vi "ex_getDaqmxChannelPropertiesCore.vi"(6 "channel props":T1[](array[typedef]), 7 "String":string, 8 "error in (no error)":errorcluster, 9 "property names (manual)":string[](array[string]), 10 "property names (autofill)":string[](array[string]), 11 "DAQmx Task":refnum<k21>) -> (0 "error out":errorcluster, 1 "Array 2":string[][](array[string]), 3 "Array":T1[][](array[typedef]))   [LabVIEW 2017]
uses:
  <vilib>/express/express shared/ex_EditUserDefinedProperties/usiDataType.ctl
  <vilib>/express/express shared/ExFile.llb/ex_TdmProperty.ctl
  <resource>/objmgr/daqmx.rc
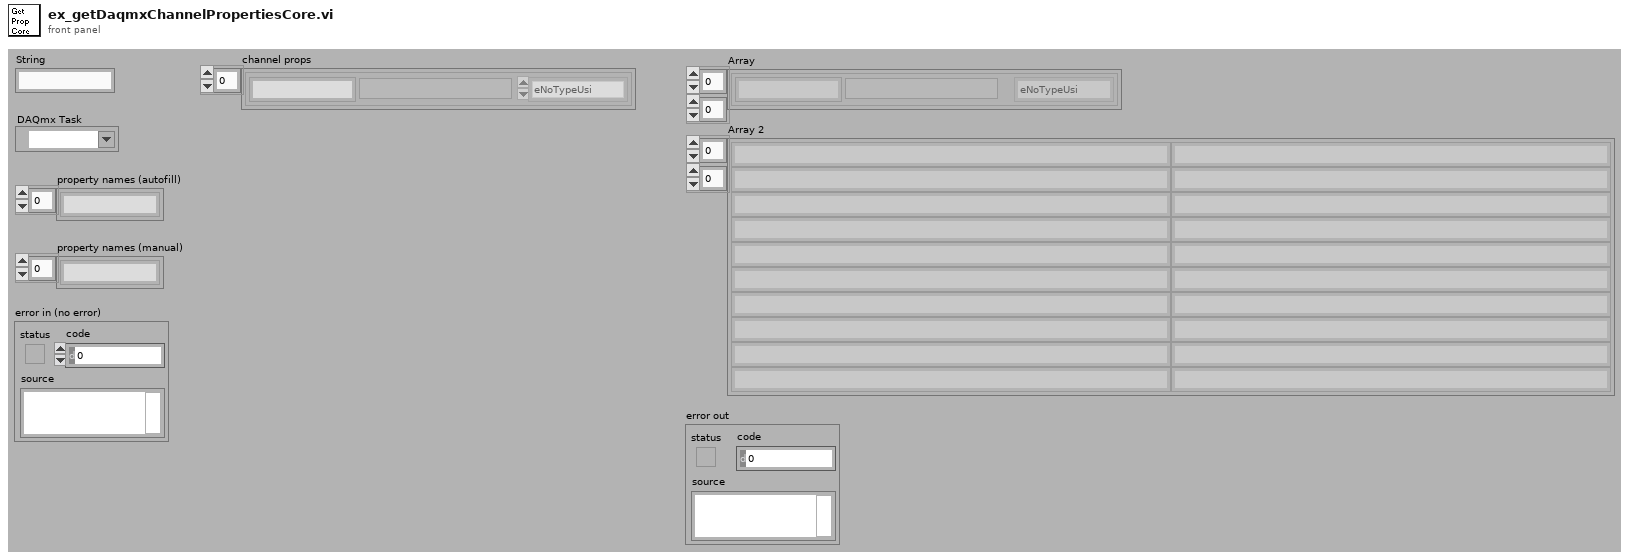
[diagram p1: front panel]
types:
  T1 = typedef "ex_TdmProperty.ctl" = cluster{"Name":string, "Type":T2, "Value":variant}
  T2 = typedef "usiDataType.ctl" = enum16{"eNoTypeUsi", "eInt8Usi", "eInt16Usi", "eInt32Usi", "eInt64Usi", "eUInt8Usi", "eUInt16Usi", "eUInt32Usi", "eUInt64Usi", "eFloat32Usi", "eFloat64Usi", "- 0", "- 1", "- 2", "- 3", "- 4", "- 5", "- 6", "- 7", "- 8", "- 9", "eString8Usi", "eString16Usi", "eStringUsi", "eEnumUsi", "- 10", "- 11", "- 12", "- 13", "- 14", "eTimeUsi", "- 15", "- 16", "- 17", "- 18", "- 19", "- 20", "- 21", "- 22", "- 23", "eInstanceUsi", "eStoreUsi"}
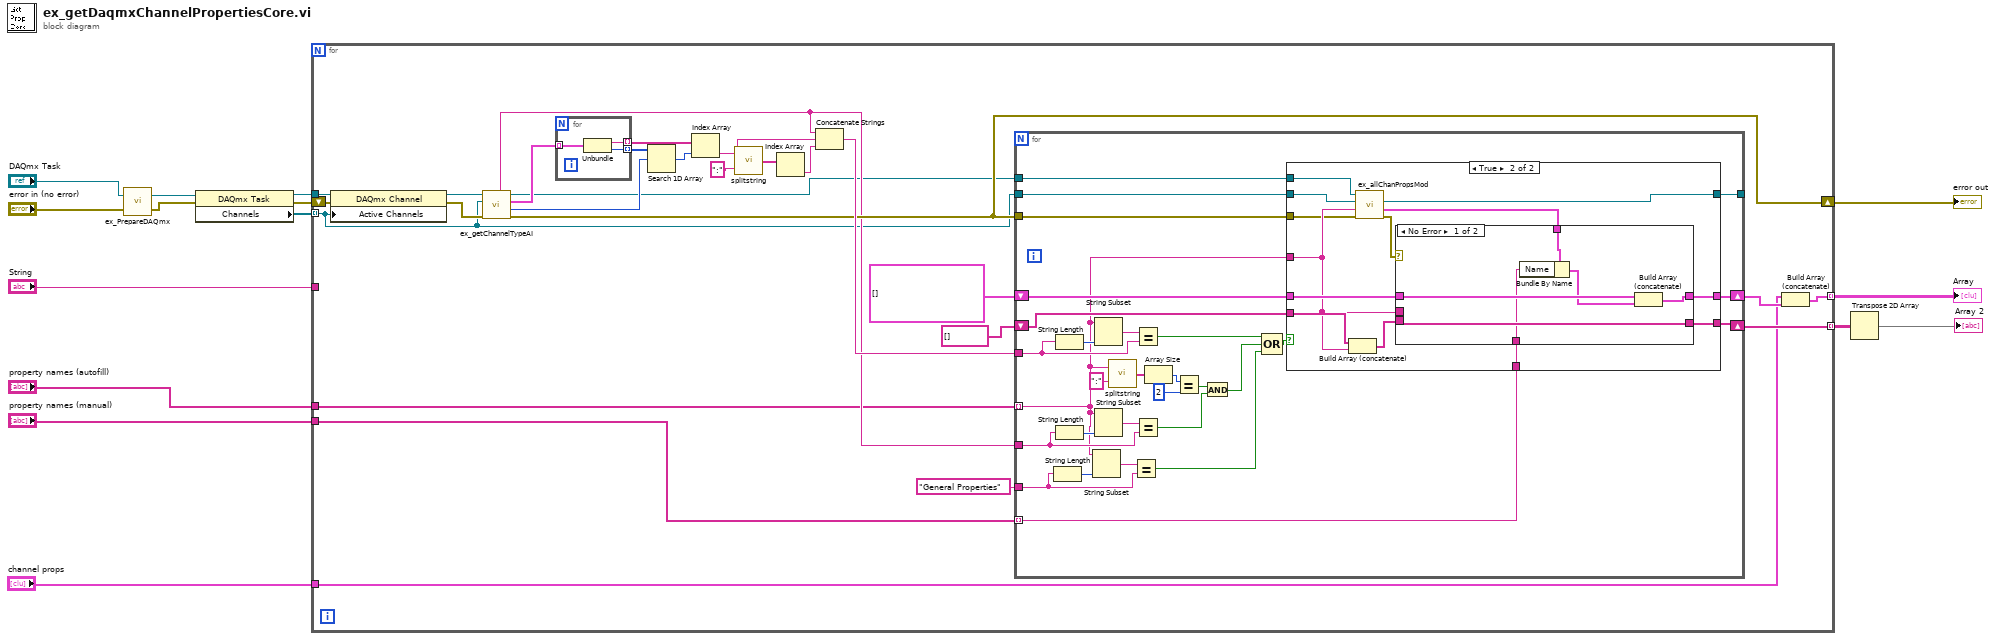
[diagram p0: block diagram]
diagram:
  n1 = call <vilib>:"ex_PrepareDAQmx.vi"("error in"="error in (no error)", "task/channels in"="DAQmx Task") -> ("error out"=w1:errorcluster, "task out"=w2:refnum<k21>)
  n2 = property class="DAQmx Task"(reference=w2, error in=w1) -> (reference out=w10:refnum<k21>, error out=w9:errorcluster, "Channels"=w15:refnum<k21>[])
  n3 = for {
    tunnel: "String" -> [_]
    tunnel: [w19] -> w13 mode=indexing
    tunnel: w15 -> [w17] mode=indexing
    tunnel: w10 -> [w42]
    tunnel: [w39] -> w11 mode=indexing
    shift-right: [w27] -> w14
    shift-left: w9 -> [w28]
    tunnel: "property names (autofill)" -> [w22]
    tunnel: "property names (manual)" -> [w21]
    tunnel: "channel props" -> [w18]
    w31 = ":" ("search string/char (-)")
    n4 = property class="DAQmx Channel"(reference=w42, error in=w28, "Active Channels"=w17) -> (reference out=w16:refnum<k21>, error out=w29:errorcluster)
    n5 = call <vilib>:"ex_getChannelTypeAI.vi"("error in (no error)"=w29, "DAQmx Global Channel"=w17, "task out"=w16) -> ("error out"=w27:errorcluster, "sub type"=w30:i32, "subsubtypes"=w35:cluster{"String":string, "Value":i32}[], "dup task"=w24:refnum<k21>, "channel type"=w25:string)  [unwired: 4 in]
    n6 = for {
      tunnel: w35 -> [w98] mode=indexing
      tunnel: [w97] -> w38 mode=indexing
      tunnel: [w96] -> w37 mode=indexing
      n7 = Unbundle(w98) -> ("String"=w96:string, "Value"=w97:i32)
    }
    n8 = Search 1D Array(1D array=w38, element=w30) -> (index of element=w36:i32)  [unwired: 1 in]
    n9 = Index Array(array=w37, index=w36) -> (element=w34:string)
    n10 = call <vilib>:"splitstring.vi"("search string/char (-)"=w31, "string"=w34) -> ("Array"=w26:string[])
    n11 = Index Array(array=w26) -> (element=w33:string)  [unwired: 1 in]
    n12 = Concatenate Strings(w25, w31, w33) -> (w32:string)
    n13 = for {
      shift-right: [w68] -> w20
      shift-left: T1[] [] -> [w69]
      shift-right: [w67] -> w39
      shift-left: string[] [] -> [w66]
      tunnel: w32 -> [w65]
      tunnel: w27 -> [w63]
      tunnel: w25 -> [w53]
      tunnel: w24 -> [w49]
      tunnel: w17 -> [w71]
      tunnel: [w70] -> _
      tunnel: "General Properties" ("channel type") -> [w48]
      tunnel: w22 -> [w44] mode=indexing
      tunnel: w21 -> [w43] mode=indexing
      n14 = String Length(string=w48) -> (length=w47:i32)
      n15 = String Length(string=w65) -> (length=w64:i32)
      n16 = String Length(string=w53) -> (length=w54:i32)
      n17 = String Subset(string=w44, length (rest)=w47) -> (substring=w46:string)  [unwired: 1 in]
      n18 = String Subset(string=w44, length (rest)=w64) -> (substring=w61:string)  [unwired: 1 in]
      n19 = String Subset(string=w44, length (rest)=w54) -> (substring=w55:string)  [unwired: 1 in]
      n20 = call <vilib>:"splitstring.vi"("search string/char (-)"=":", "string"=w44) -> ("Array"=w60:string[])
      n21 = Equal?(x=w46, y=w48) -> (x = y?=w45:bool)
      n22 = Equal?(x=w61, y=w65) -> (x = y?=w58:bool)
      n23 = Equal?(x=w55, y=w53) -> (x = y?=w51:bool)
      n24 = Array Size(array=w60) -> (size(s)=w59:i32)
      n25 = Equal?(x=w59, y=2) -> (x = y?=w52:bool)
      n26 = And(x=w52, y=w51) -> (x .and. y?=w50:bool)
      n27 = Compound Arithmetic op=OR(w58, w50, w45) -> (w57:bool)
      n28 = case shown="True" w57 {
        tunnel: w71 -> [w73 w87]
        tunnel: [w73 w86] -> w70
        tunnel: w44 -> [_ w79]
        tunnel: w69 -> [w74 w85]
        tunnel: [w74 w84] -> w68
        tunnel: [w72 w81] -> w67
        tunnel: w66 -> [w72 w80]
        tunnel: w63 -> [_ w77]
        tunnel: w49 -> [_ w76]
        tunnel: w43 -> [_ w75]
        frame False {
        }
        frame True {
          n29 = Build Array (concatenate)(w80, w79) -> (w78:string[])
          n30 = call <vilib>:"ex_allChanPropsMod.vi"("error in (no error)"=w77, "propertySource"=w79, "DAQmx Channel"=w87, "DAQmx Task"=w76) -> ("error out"=w82:errorcluster, "TDM Property"=w83:T1, "dup DAQmx Channel"=w86:refnum<k21>)  [unwired: 1 in]
          n31 = case shown="No Error" w82 {
            tunnel: w85 -> [w93 w95]
            tunnel: [w92 w95] -> w84
            tunnel: w83 -> [w90 _]
            tunnel: w79 -> [_ _]
            tunnel: [w91 w94] -> w81
            tunnel: w78 -> [w91 w94]
            tunnel: w75 -> [w88 _]
            frame No Error {
              n32 = Bundle By Name(cluster=w90, "Name"=w88) -> (w89:T1)
              n33 = Build Array (concatenate)(w93, w89) -> (w92:T1[])
            }
            frame Error {
            }
          }
        }
      }
    }
    n34 = Build Array (concatenate)(w18, w20) -> (w19:T1[])
  }
  "error out" <- w14
  "Array" <- w13
  n35 = Transpose 2D Array(2D array=w11) -> (transposed array=→"Array 2":string[][])
